vi "niSE_Close.vi"(8 "error in":errorcluster {"code" format="%.0x"}, 11 "Handle":variant) -> (0 "error out":errorcluster {"code" format="%.0x"})   [LabVIEW 2015]
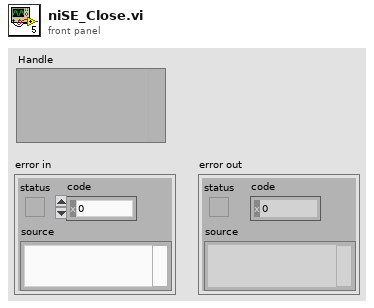
[diagram p1: front panel]
types:
  T1 = typedef "niSE SessionRefnum.ctl" = refnum<k1>
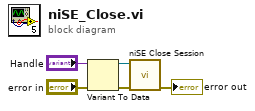
[diagram p0: block diagram]
diagram:
  n1 = Variant To Data(error in="error in", Variant="Handle") -> (data=w3:T1, error out=w2:errorcluster)  [unwired: 1 in]
  n2 = call <vilib>:"niSE Close Session.vi"("error in (no error)"=w2, "NISE Session (in)"=w3) -> ("error out"=→"error out":errorcluster)  [unwired: 5 in]
